vi "Is Created Event.vi"(10 "Created Event Alias":string, 11 "Base Queue in":refnum<class "Base Queue.lvclass">) -> (2 "Is Created Event?":bool, 3 "Base Queue out":refnum<class "Base Queue.lvclass">)   [LabVIEW 2021, in "jettl.lvlib" / "Base Queue.lvlib" / "Base Queue.lvclass"]
uses:
  Base Queue.lvclass
  C:/git/jettl/src/jettl/jettl/jettl.lvclass
  Base Queue.lvclass/Base Queue.ctl
  Queue Mailbox/Queue Mailbox.lvlib
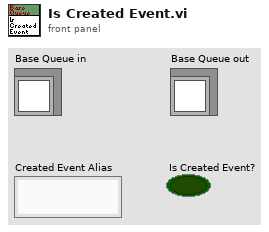
[diagram p1: front panel]
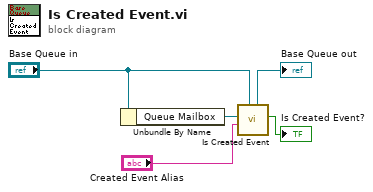
[diagram p0: block diagram]
diagram:
  n1 = Unbundle By Name("Base Queue in") -> ("Queue Mailbox"=w5:refnum<data-value>)
  n2 = call "Is Created Event.vi"("jettl in"="Base Queue in", "Created Event Alias"="Created Event Alias", "Queue Mailbox"=w5) -> ("Is Created Event?"=→"Is Created Event?":bool, "jettl out"=→"Base Queue out":refnum<class "Base Queue.lvclass">)  [unwired: 7 in]
